vi "EXCEL READ AND WRITE.vi"(0 "Automation Refnum in":refnum<k7>, 1 "CELL":string, 2 "SHEET INDEX":dbl, 5 "Excel.Application REF in":refnum<k7>, 7 "Excel._Workbook":refnum<k7>, 13 "OPERATION":enum16{"READ", "WRITE"}(ring), 14 "STRING TO WRITE":string) -> (4 "Excel Application ref out":refnum<k7>, 6 "WORKBOOK REF OUT":refnum<k7>, 8 "READING FROM EXCEL":string)   [LabVIEW 2021]
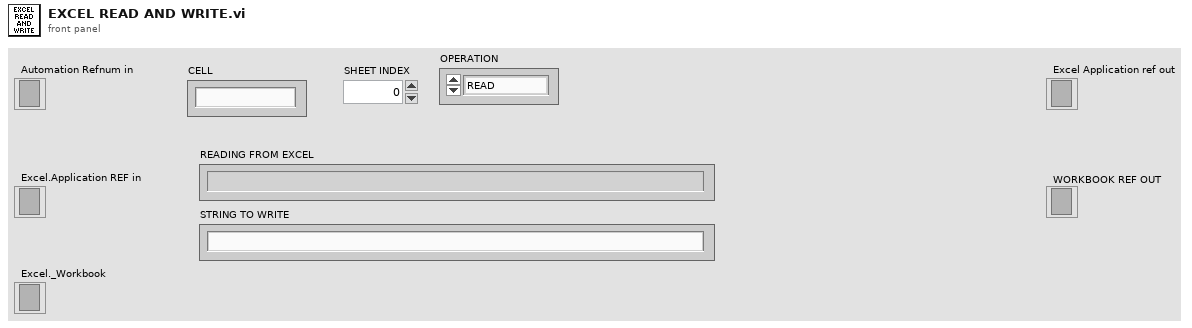
[diagram p1: front panel]
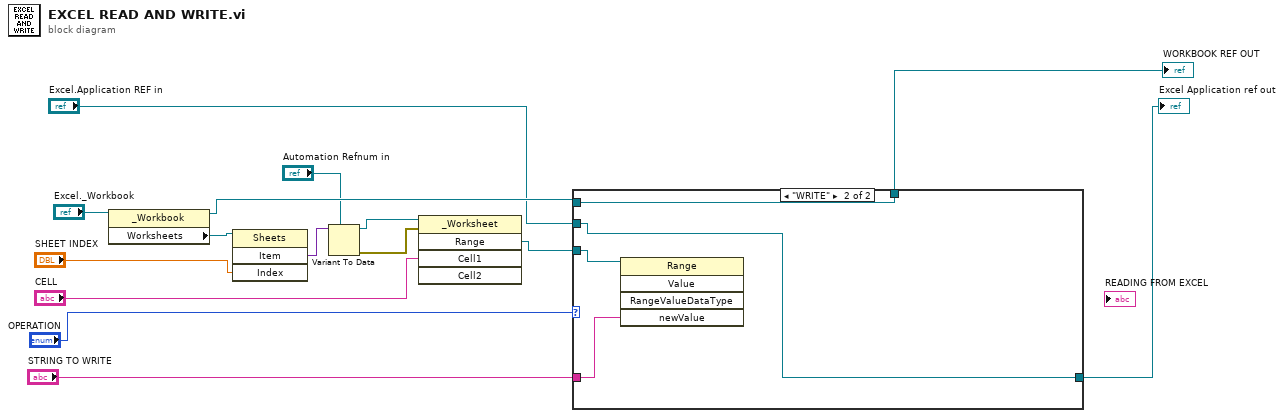
[diagram p0: block diagram]
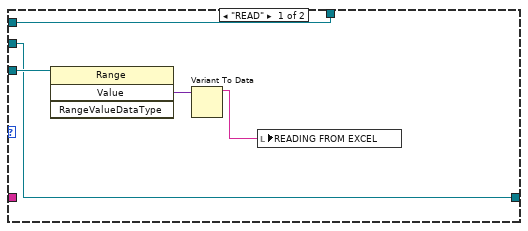
[diagram p2: hidden frame]
diagram:
  n1 = property class="_Workbook"(reference="Excel._Workbook") -> (reference out=w14:refnum<k7>, "Worksheets"=w3:refnum<k7>)  [unwired: 1 in, 1 out]
  n2 = invoke class="Sheets" method="Item"(reference=w3, "Index"="SHEET INDEX") -> ("Item"=w5:variant)  [unwired: 2 in, 3 out]
  n3 = Variant To Data(type="Automation Refnum in", Variant=w5) -> (data=w1:refnum<k7>, error out=w7:errorcluster)  [unwired: 1 in]
  n4 = invoke class="_Worksheet" method="Range"(reference=w1, error in=w7, "Cell1"="CELL") -> ("Range"=w10:refnum<k7>)  [unwired: 2 in, 4 out]
  n5 = case shown="\"WRITE\"" "OPERATION" {
    tunnel: w10 -> [w20 w22]
    tunnel: "STRING TO WRITE" -> [_ w21]
    tunnel: "Excel.Application REF in" -> [w18 w24]
    tunnel: [w18 w24] -> w13
    tunnel: w14 -> [w17 w23]
    tunnel: [w17 w23] -> w15
    frame "READ" {
      n6 = invoke class="Range" method="Value"(reference=w20) -> ("Value"=w19:variant)  [unwired: 3 in, 3 out]
      n7 = Variant To Data(Variant=w19) -> (data=w16:string)  [unwired: 2 in, 1 out]
      n8 = local write "READING FROM EXCEL"(w16) -> ()
    }
    frame "WRITE" {
      n9 = invoke class="Range" method="Value"(reference=w22, "newValue"=w21) -> ()  [unwired: 3 in, 5 out]
    }
  }
  "Excel Application ref out" <- w13
  "WORKBOOK REF OUT" <- w15
